vi "Init_StringAccumulator.vi"() -> (3 "Accumulator":refnum<class "Accumulator.lvclass">)   [LabVIEW 2020, in "Accumulator.lvclass"]
uses:
  Accumulator.lvclass
  Accumulator.lvclass/Accumulator.ctl
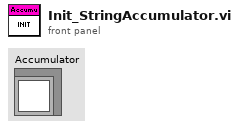
[diagram p1: front panel]
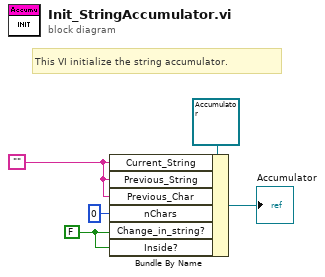
[diagram p0: block diagram]
diagram:
  w2 = FALSE ("Change_in_string?")
  w4 = ""
  # "This VI initialize the string accumulator."
  n1 = Bundle By Name(cluster=refnum<class "Accumulator.lvclass"> refnum ("Accumulator.lvclass"), "Current_String"=w4, "Previous_String"=w4, "Previous_Char"=w4, "nChars"=0, "Change_in_string?"=w2, "Inside?"=w2) -> (→"Accumulator":refnum<class "Accumulator.lvclass">)
